vi "Test_DT1.vi"() -> ()   [LabVIEW 2022 SP3]
uses:
  <vilib>/measure/NI_MABase.lvlib
panel:
  out "XY Graph":cluster{dbl[], dbl[]}(graph)
  in  "sampling info":cluster{"Fs":dbl, "#s":dbl}={"Fs"=1000.0, "#s"=1000.0} {"Fs" format="%.2p"}
  in  "initialize":bool
  in  "T1":dbl
  in  "G":dbl
  in  "amplitude":dbl=1.0 format="%0.2p"
  in  "frequency":dbl=10.0 format="%0.2p"
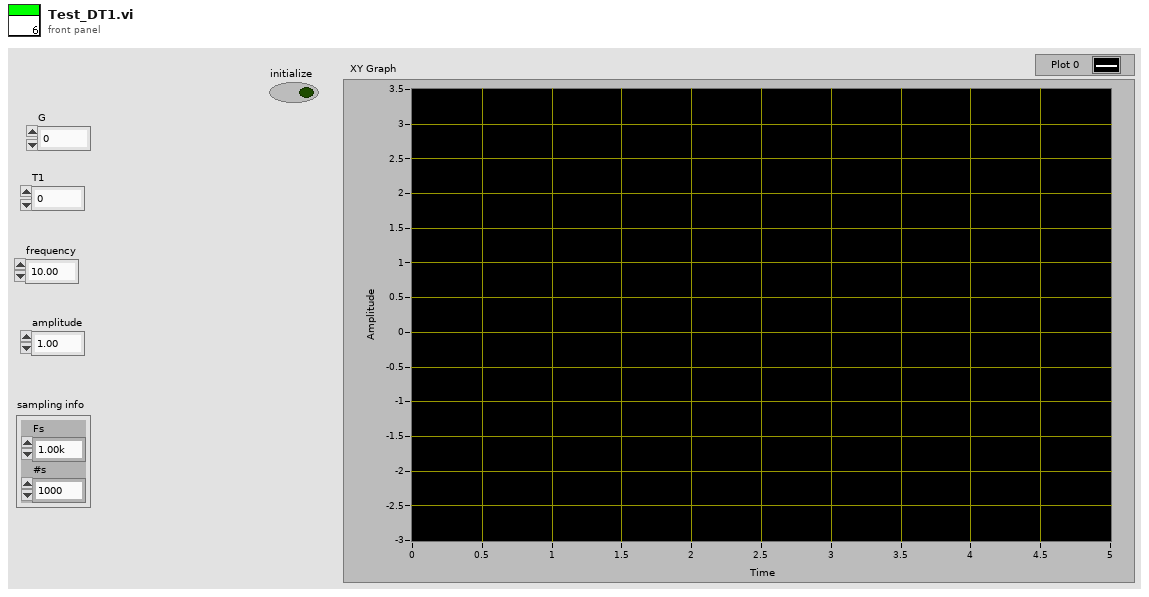
[diagram p1: front panel]
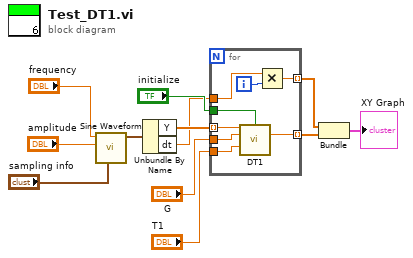
[diagram p0: block diagram]
diagram:
  n1 = call <vilib>:"Sine Waveform.vi"("sampling info"="sampling info", "amplitude"="amplitude", "frequency"="frequency") -> ("signal out"=w10:waveform(dbl))  [unwired: 7 in, 1 out]
  n2 = Unbundle By Name(w10) -> ("Y"=w9:dbl[], "dt"=w5:dbl)
  n3 = for {
    tunnel: w9 -> [w17] mode=indexing
    tunnel: "G" -> [w15]
    tunnel: "T1" -> [w14]
    tunnel: "initialize" -> [w16]
    tunnel: w5 -> [w19]
    tunnel: [w18] -> w3 mode=indexing
    tunnel: [w13] -> w2 mode=indexing
    i -> [w20]
    n4 = call "DT1.vi"("input u(k)"=w17, "initialize"=w16, "G"=w15, "T1"=w14) -> ("output y(k)"=w13:dbl)  [unwired: 10 in, 1 out]
    n5 = Multiply(x=w19, y=w20) -> (x*y=w18:dbl)
  }
  n6 = Bundle(w3, w2) -> (→"XY Graph":cluster{dbl[], dbl[]})  [unwired: 1 in]
